vi "main.vi"() -> ()   [LabVIEW 2017]
uses:
  <vilib>/Platform/TimedLoop/XDataNode/wakeup.ctl
  <vilib>/Platform/TimedLoop/XDataNode/XDNodeRunTimeDep.lvlib
  <vilib>/Platform/TimedLoop/XDataNode/nitl_modes.ctl
  <vilib>/Platform/TimedLoop/XDataNode/timing_clust.ctl
  <vilib>/Platform/TimedLoop/XDataNode/XDataNode.xnode
  <vilib>/xnet/xnet.llb/XNET Frame Type CAN.ctl
  <vilib>/xnet/xnet.llb/XNET Frame CAN.ctl
  <vilib>/rvi/interface/nirviReadWriteControl/nirviReadWriteControl.xnode
  FPGA Bitfiles/FPGA.ctl
  FPGA Bitfiles/PVemulator_FPGATarget2_IpDFT-only-DC2x9_aEit3VyAdvg.lvbitx
  <vilib>/xnet/xnet.llb/XNET Write (Frame CAN).vi
  <vilib>/xnet/xnet.llb/XNET Read (Frame CAN).vi
  NiFpgaLv.dll
  <vilib>/Utility/error.llb/Error Cluster From Error Code.vi
  <vilib>/rvi/errors/niLvFpgaAdjustHostInterfaceError.vi
  General purpose/measurements.ctl
panel:
  out "Numeric":i32
  in  "Meas":T1
  out "V_PV1":dbl
  out "Ok to Close Contactor":bool
  out "CAN frame":T2 {"payload" format="%x"; "timestamp" format="%<%.7X\n%x>T"; "type" items=["CAN Data"=0, "CAN Remote"=1, "CAN Bus Error"=2, "CAN 2.0 Data"=8, "CAN FD Data"=16, "CAN FD+BRS Data"=24, "J1939 Data"=192, "Delay"=224, "Log Trigger"=225, "Start Trigger"=226]; "identifier" format="%x"}
  out "Vdc DCLink":dbl
  out "RPi Monitoring":bool
  out "Pconv":dbl
  out "Alarm list":string
  in  "Meas period [ms]":i64=10
  in  "newfile":bool
  in  "Log period [ms]":i64=1000
  out "Con_State":u8(ring) items=["Idle"=0, "Busy"=1, "Wait4srcON"=2, "Ready"=3, "Injecting"=6]
  in  "Emergency":bool
  in  "p_sp":dbl
  in  "Conv":T4
  in  "CAN [ms]":i64=1
  out "full":bool
  out "neg":bool
  out "precharge":bool
  out "CAN with Conv":bool
  out "Measurements":bool
  in  "Shutdwn":bool
  in  "Clear":bool
  in  "SEND sp":bool
  in  "Start":bool
  out "Error":u8(ring) items=["None", "Converter (water/temp/desat)", "Overvalue (hardware detected)", "Internal DC bus low", "Internal DC bus high", "External source DC low", "External source DC high", "Grid present (while VSC)", "Grid voltage out of range", "Grid frequency out of range", "No Grid (while CSC)", "Cannot clear (Manual clear needed)", "User Emergency", "Latch-up (Restart BBX)"]
  out "logging":bool
  in  "main stop":bool
  # "Resource agent: PV emulator x2 + Battery"
  # "PV Emulator for a DC grid"
  # "package identifiers:\n1xx PV emulator\n2xx PV emulator\n3xx PV emulator \n4xx battery\n\nx0x send from agent to resource\nx00 Power setpoints\nx01 Measurements\nx02 status\n          = [0; clear; 0; 0; 0; off; emergence; start]\n\n \n\nx1x send from resource to agent\nx10 Power measurements\nx11 Measurements\nx12 status\n          = [state; error; alarm; full; precharge; neg; 0; 0]"
  # "State:"
  # "DC +"
  # "DC -"
  # "CONVERTER CONTROL"
  # "PV"
  # "SETPOINTS"
  # "DC"
  # "DC"
  # "R"
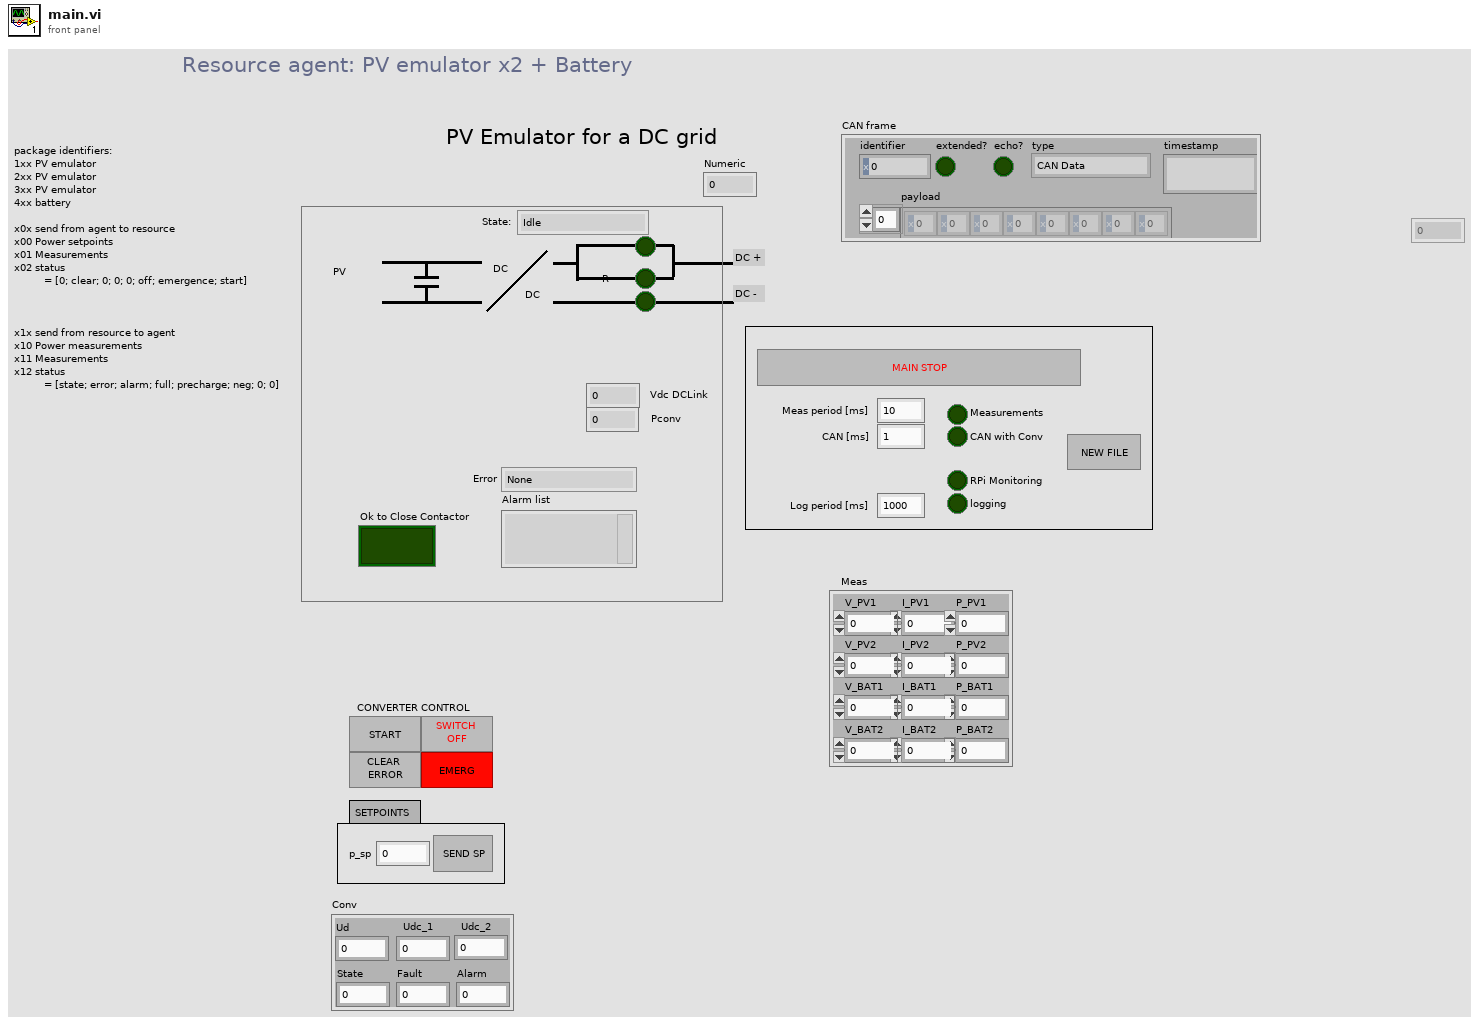
[diagram p1: front panel]
types:
  T1 = typedef "measurements.ctl" = cluster{"V_PV1":dbl, "I_PV1":dbl, "V_PV2":dbl, "I_PV2":dbl, "P_PV2":dbl, "V_BAT1":dbl, "I_BAT1":dbl, "P_BAT1":dbl, "V_BAT2":dbl, "I_BAT2":dbl, "P_BAT2":dbl, "P_PV1":dbl}
  T2 = typedef "XNET Frame CAN.ctl" = cluster{"timestamp":timestamp, "payload":u8[], "identifier":u32, "type":T3, "extended?":bool, "echo?":bool}
  T3 = typedef "XNET Frame Type CAN.ctl" = u8
  T4 = cluster{"Ud":dbl, "State":dbl, "Fault":dbl, "Alarm":dbl, "Udc_1":dbl, "Udc_2":dbl}
  T5 = typedef "FPGA.ctl" = refnum<k20>
  T6 = cluster{"Frame In":refnum<k21>, "Frame Out":refnum<k21>}
  T7 = typedef "XDNodeRunTimeDep.lvlib/timing_clust.ctl" = cluster{"Expected End [f-1]":u64, "Actual End [f-1]":u64, "Finished Late? [f-1]":bool, "Expected End [i-1]":u64, "Actual End [i-1]":u64, "Finished Late? [i-1]":bool, "Expected Start [i]":u64, "Actual Start [i]":u64, "Expected Start [f]":u64, "Actual Start [f]":u64, "Source Name":string, "Structure Name":string, "Period":i64, "Deadline":i64, "Offset":i64, "Start":i64, "Priority":i32, "Timeout":i32, "Mode":T8, "Wakeup Reason":T9, "Error":errorcluster, "Source Type":string, "Secondary Source Type":string, "Global End Time":u64, "Global Start Time":u64, "Frame Duration":u64, "Iteration Duration":u64, "Assigned CPU":i32, "I/O Scan Engine Mode":u32}
  T8 = typedef "XDNodeRunTimeDep.lvlib/nitl_modes.ctl" = enum32{"No Change", "Process missed periods, maintain original phase", "Discard missed periods, maintain original phase", "Process missed periods, ignore original phase", "Discard missed periods, ignore original phase"}
  T9 = typedef "XDNodeRunTimeDep.lvlib/wakeup.ctl" = enum32{"Normal", "Aborted", "Asynchronous wakeup", "Timing source error", "Timed loop error", "Timeout"}
  T10 = cluster{"V_PV1":dbl, "I_PV1":dbl, "V_PV2":dbl, "I_PV2":dbl, "P_PV2":dbl, "V_BAT1":dbl, "I_BAT1":dbl, "P_BAT1":dbl, "V_BAT2":dbl, "I_BAT2":dbl, "P_BAT2":dbl, "P_PV1":dbl}
  T11 = cluster{"date string":string, "time string":string, "V_PV1":dbl, "I_PV1":dbl, "P_PV1":dbl, "V_PV2":dbl, "I_PV2":dbl, "P_PV2":dbl, "V_BAT1":dbl, "I_BAT1":dbl, "P_BAT1":dbl, "V_BAT2":dbl, "I_BAT2":dbl, "P_BAT2":dbl}
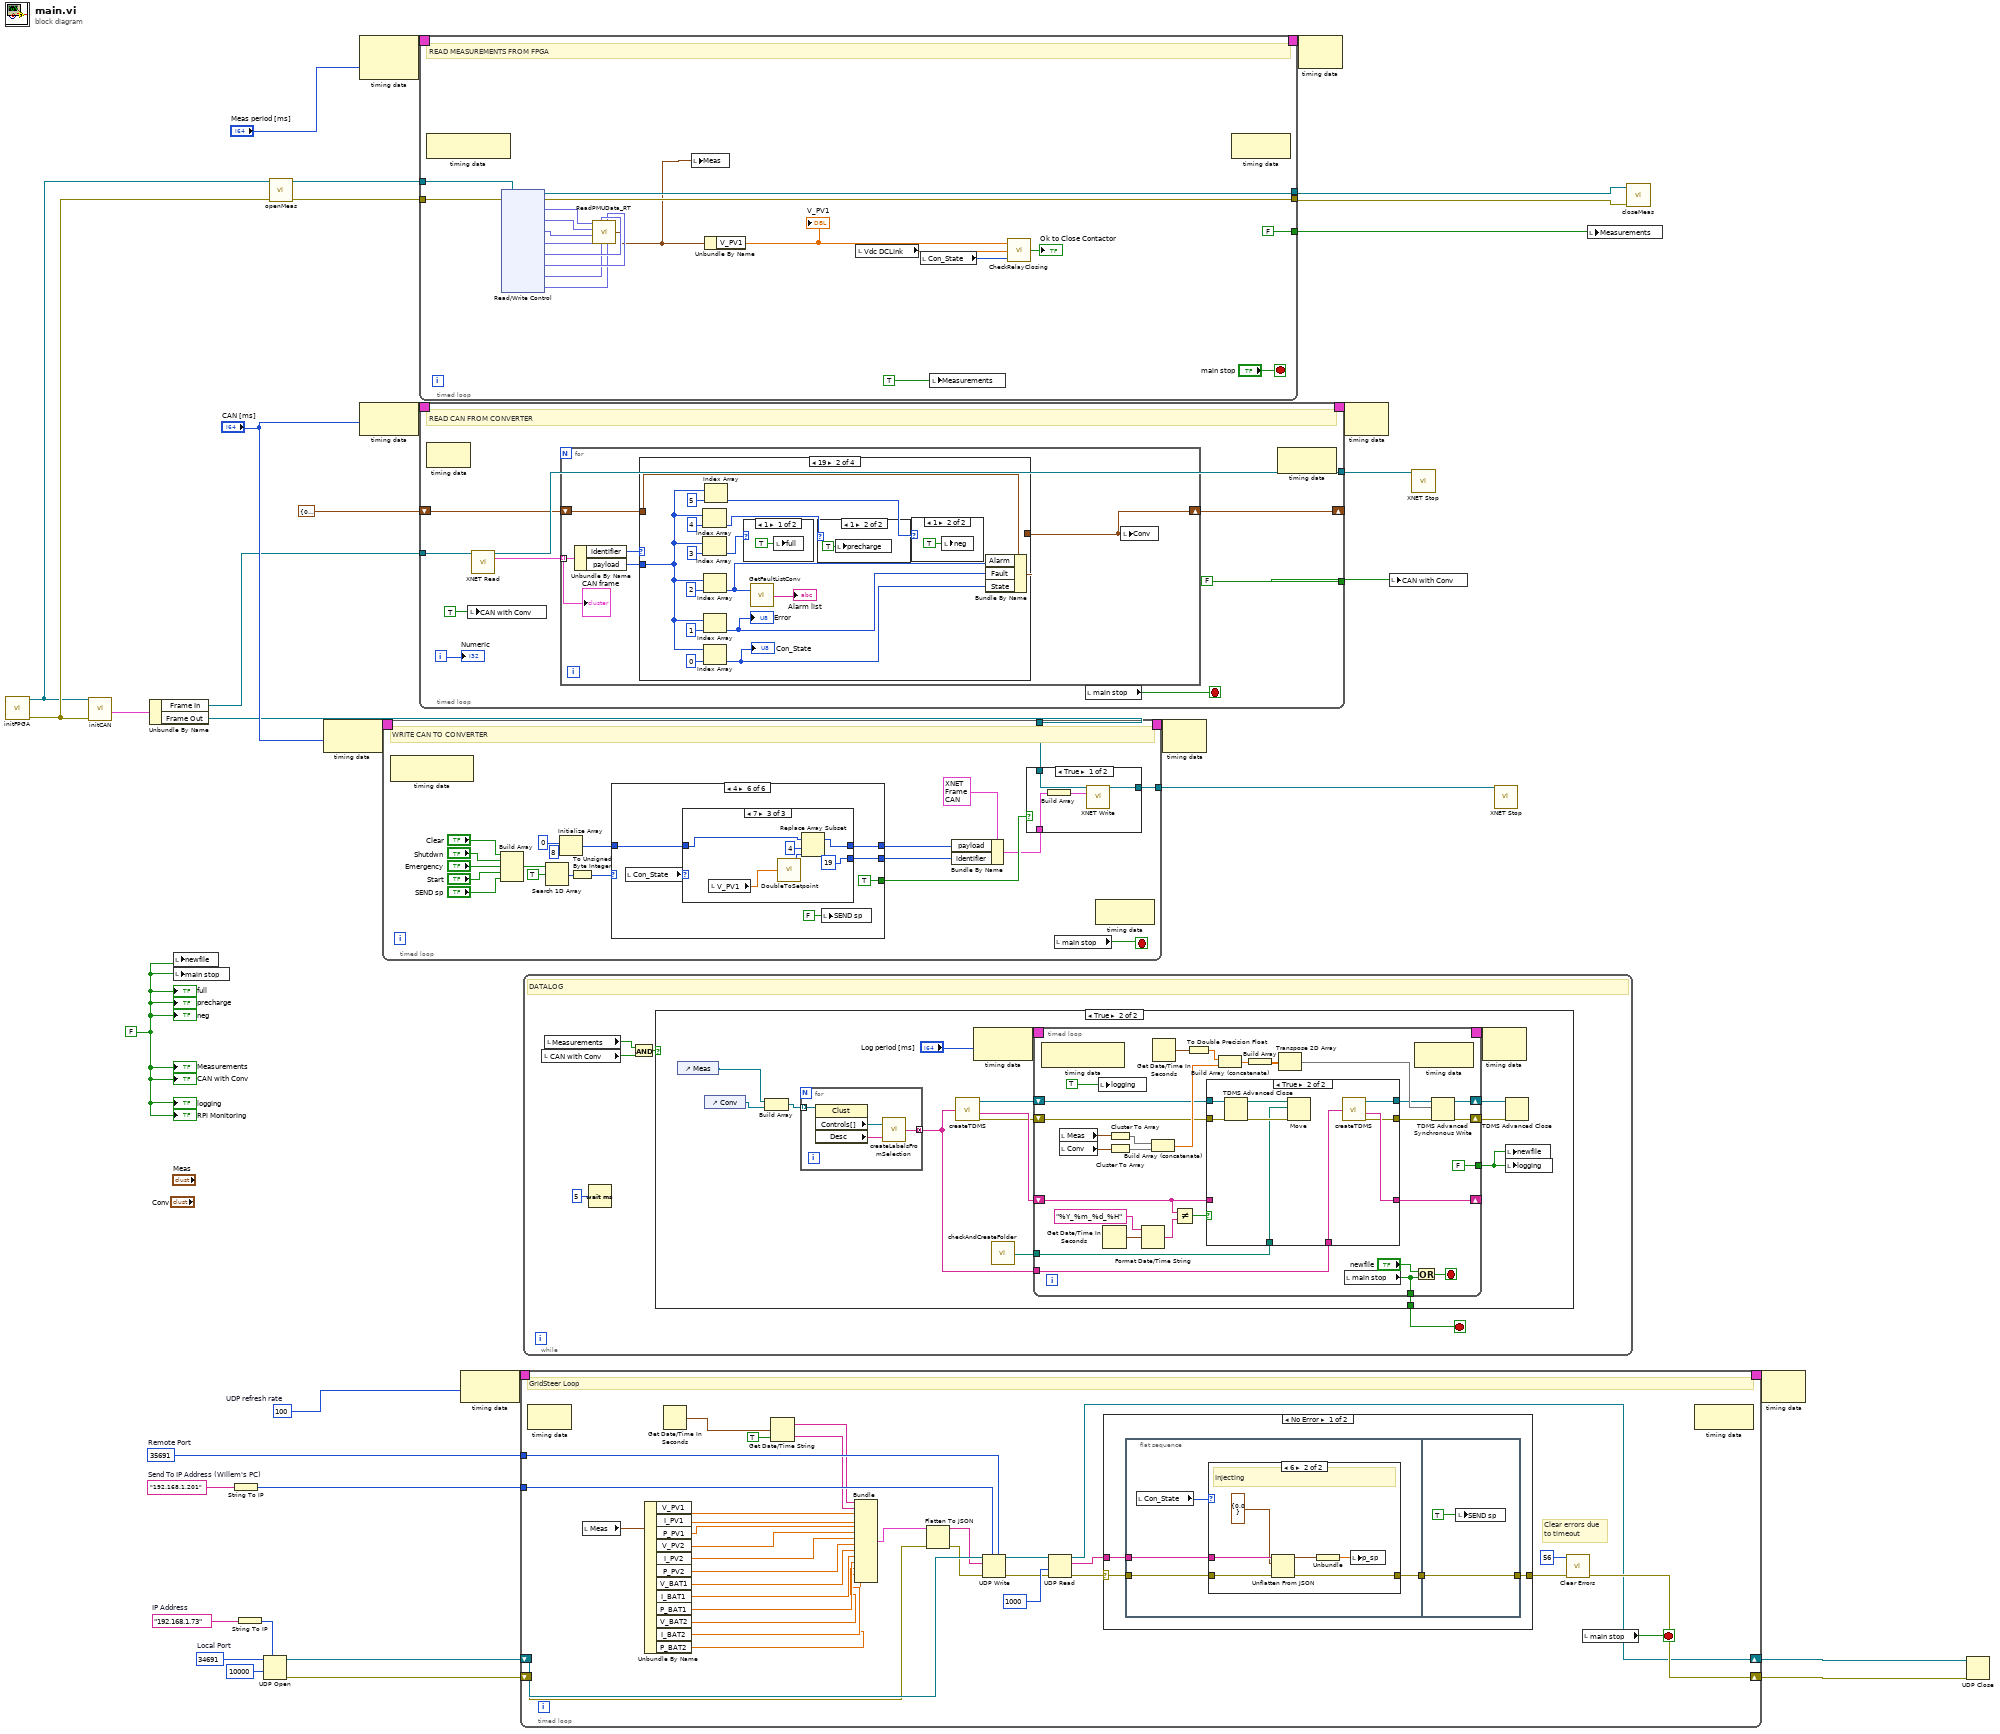
[diagram p0: block diagram]
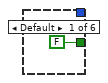
[diagram p7: hidden frame]
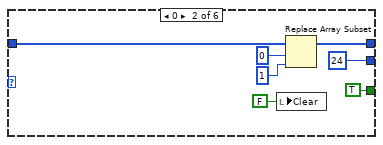
[diagram p8: hidden frame]
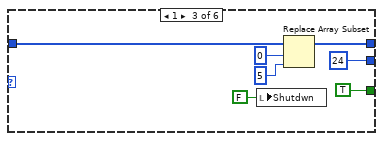
[diagram p9: hidden frame]
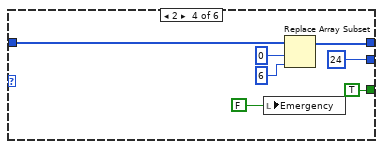
[diagram p10: hidden frame]
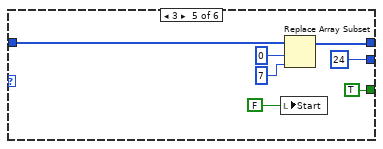
[diagram p11: hidden frame]
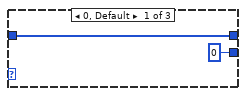
[diagram p12: hidden frame]
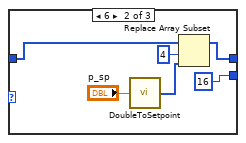
[diagram p13: hidden frame]
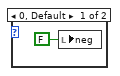
[diagram p15: hidden frame]
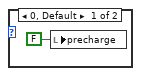
[diagram p16: hidden frame]
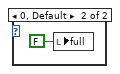
[diagram p17: hidden frame]
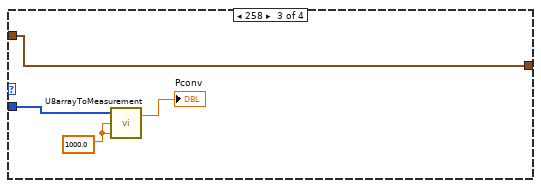
[diagram p18: hidden frame]
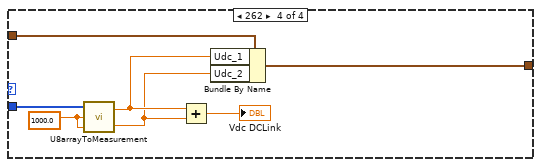
[diagram p19: hidden frame]
diagram:
  w5 = i64 100  # UDP refresh rate
  w10 = u16 34691  # Local Port
  w11 = "192.168.1.73"  # IP Address
  w1 = u16 35691  # Remote Port
  w9 = "192.168.1.201"  # Send To IP Address (Willem's PC)
  w17 = FALSE
  n1 = call "initFPGA.vi"() -> ("FPGA VI Reference Out"=w16:T5, "error out"=w18:errorcluster)  [unwired: 4 in]
  n2 = call "initCAN.vi"("error in"=w18, "FPGA VI (in)"=w16) -> ("CAN"=w31:T6)  [unwired: 3 in, 2 out]
  n3 = Unbundle By Name(w31) -> ("Frame In"=w21:refnum<k21>, "Frame Out"=w20:refnum<k21>)
  n4 = local write "newfile"(w17) -> ()
  n5 = local write "main stop"(w17) -> ()
  n6 = String To IP(1:w9) -> (0:w2:u32)
  n7 = String To IP(1:w11) -> (0:w12:u32)
  n8 = UDP Open(7:w12, 9:10000 ("timeout ms (25000)"), 11:w10) -> (port=w4:refnum<k16>, 0:w3:errorcluster)  [unwired: 2 in, 1 out]
  n9 = call "openMeas.vi"("error in"=w18, "FPGA VI (in)"=w16) -> ("error out"=w25:errorcluster, "FPGA VI (out)"=w26:T5)  [unwired: 7 in, 1 out]
  n10 = node-c288("CAN [ms]") -> (w33:T7)
  n11 = node-c288("Meas period [ms]") -> (w37:T7)  [unwired: 1 in]
  n12 = node-c288("CAN [ms]") -> (w35:T7)
  n13 = timed-loop {
    tunnel: w20 -> [w49]
    tunnel: [w48] -> w29
    timing: w33 -> [_]
    timing-out: [_] -> w32
    stop <- w47 stop-if-true
    # "WRITE CAN TO CONVERTER"
    n14 = node-c288() -> ()  [unwired: 1 in, 1 out]
    n15 = Build Array("Clear", "Shutdwn", "Emergency", "Start", "SEND sp") -> (w46:bool[])
    n16 = Search 1D Array(1D array=w46, element=TRUE) -> (index of element=w40:i32)  [unwired: 1 in]
    n17 = Initialize Array(u8 0, 8 ("dimension size")) -> (w55:u8[])
    n18 = To Unsigned Byte Integer(number=w40) -> (unsigned 8bit integer=w44:u8)
    n19 = case shown="4" w44 {
      tunnel: [_ w70 w77 w83 w90 w98] -> w54
      tunnel: [_ u32 24 ("identifier") u32 24 ("identifier") u32 24 ("identifier") u32 24 ("identifier") w95] -> w53
      tunnel: w55 -> [_ w68 w76 w84 w91 w93]
      tunnel: [FALSE TRUE TRUE TRUE TRUE TRUE] -> w51
      frame Default {
      }
      frame 0 {
        n20 = local write "Clear"(FALSE ("Clear")) -> ()
        n21 = Replace Array Subset(array=w68, new element=u8 1 ("new element/subarray"), index=0) -> (w70:u8[])
      }
      frame 1 {
        n22 = local write "Shutdwn"(FALSE ("Shutdwn")) -> ()
        n23 = Replace Array Subset(array=w76, new element=u8 5 ("new element/subarray"), index=0) -> (w77:u8[])
      }
      frame 2 {
        n24 = local write "Emergency"(FALSE ("Idc cmd")) -> ()
        n25 = Replace Array Subset(array=w84, new element=u8 6 ("new element/subarray"), index=0) -> (w83:u8[])
      }
      frame 3 {
        n26 = local write "Start"(FALSE ("Idc cmd")) -> ()
        n27 = Replace Array Subset(array=w91, new element=u8 7 ("new element/subarray"), index=0) -> (w90:u8[])
      }
      frame 4 {
        n28 = local read "Con_State"() -> (w94:u8)
        n29 = case shown="7" w94 {
          tunnel: [w100 w104 w110] -> w98
          tunnel: [u32 0 ("identifier") u32 16 ("identifier") u32 19 ("identifier")] -> w95
          tunnel: w93 -> [w100 w102 w107]
          frame 0, Default {
          }
          frame 6 {
            n30 = call "DoubleToSetpoint.vi"("Double"="p_sp") -> ("SP"=w103:u8[])
            n31 = Replace Array Subset(array=w102, new element=w103, index=4) -> (w104:u8[])
          }
          frame 7 {
            n32 = local read "V_PV1"() -> (w111:dbl)
            n33 = call "DoubleToSetpoint.vi"("Double"=w111) -> ("SP"=w109:u8[])
            n34 = Replace Array Subset(array=w107, new element=w109, index=4) -> (w110:u8[])
          }
        }
        n35 = local write "SEND sp"(FALSE ("SEND sp")) -> ()
      }
    }
    n36 = Bundle By Name(cluster=T2 {"timestamp"=timestamp(0 s since 1904-01-01), "payload"=[], "identifier"=0, "type"=0, "extended?"=FALSE, "echo?"=FALSE} ("CAN frame 3"), "payload"=w54, "identifier"=w53) -> (w50:T2)
    n37 = case shown="True" w51 {
      tunnel: w50 -> [w63 _]
      tunnel: w49 -> [w61 _]
      tunnel: [w60 _] -> w48
      frame True {
        n38 = Build Array(w63) -> (w62:T2[])
        n39 = call-poly <vilib>:"XNET Write.vi"("session in"=w61, "data"=w62) -> ("session out"=w60:refnum<k21>)  [unwired: 12 in, 1 out]
      }
      frame False {
      }
    }
    n40 = local read "main stop"() -> (w47:bool)
    n41 = node-c288() -> ()  [unwired: 1 in, 1 out]
  }
  n42 = timed-loop {
    timing: w37 -> [_]
    timing-out: [_] -> w36
    tunnel: w26 -> [w124]
    tunnel: [w125] -> w24
    tunnel: [w126] -> w23
    tunnel: [FALSE] -> w27
    tunnel: w25 -> [w123]
    stop <- "main stop" stop-if-true
    # "READ MEASUREMENTS FROM FPGA"
    n43 = node-c288() -> ()  [unwired: 1 in, 1 out]
    n44 = xnode "Read/Write Control"("FPGA VI Reference In"=w124, "error in"=w123) -> ("FPGA VI Reference Out"=w125:T5, "error out"=w126:errorcluster, "V_PV1"=w122:fxp<+,20,5>, "I_PV1"=w121:fxp<+,20,5>, "V_PV2"=w120:fxp<+/-,20,5>, "I_PV2"=w119:fxp<+/-,20,5>, "V_BAT1"=w118:fxp<+/-,20,5>, "I_BAT1"=w117:fxp<+,20,5>, "V_BAT2"=w116:fxp<+,20,5>, "I_BAT2"=w115:fxp<+/-,20,5>)
    n45 = call "ReadPMUData_RT.vi"("I_BAT2"=w115, "I_BAT1"=w117, "V_BAT2"=w116, "I_PV2"=w119, "V_PV2"=w120, "V_BAT1"=w118, "I_PV1"=w121, "V_PV1"=w122) -> ("measurements"=w113:T10)  [unwired: 2 in]
    n46 = local write "Meas"(w113) -> ()
    n47 = Unbundle By Name(w113) -> ("V_PV1"=w114:dbl)
    "V_PV1" <- w114
    n48 = local read "Vdc DCLink"() -> (w128:dbl)
    n49 = local read "Con_State"() -> (w127:u8)
    n50 = local write "Measurements"(TRUE) -> ()
    n51 = call "CheckRelayClosing.vi"("Converter State"=w127, "Vdc DC Link"=w128, "Vdc Battery"=w114) -> ("Ok to Close Contactor"=→"Ok to Close Contactor":bool)
    n52 = node-c288() -> ()  [unwired: 1 in, 1 out]
  }
  n53 = timed-loop {
    timing: w35 -> [_]
    timing-out: [_] -> w34
    tunnel: w21 -> [w135]
    tunnel: [w142] -> w30
    shift-right: [w137] -> _
    shift-left: T4 {"Ud"=0.0, "State"=0.0, "Fault"=0.0, "Alarm"=0.0, "Udc_1"=0.0, "Udc_2"=0.0} ("Conv") -> [w141]
    tunnel: [FALSE ("stop CAN")] -> w19
    i -> [w136]
    stop <- w140 stop-if-true
    # "READ CAN FROM CONVERTER"
    n54 = node-c288() -> ()  [unwired: 1 in, 1 out]
    n55 = local write "CAN with Conv"(TRUE) -> ()
    n56 = call-poly <vilib>:"XNET Read.vi"("session in"=w135) -> ("session out"=w142:refnum<k21>, "data"=w143:T2[])  [unwired: 11 in, 2 out]
    n57 = for {
      tunnel: w143 -> [w146] mode=indexing
      shift-right: [w144] -> w137
      shift-left: w141 -> [w145]
      n58 = Unbundle By Name(w146) -> ("identifier"=w148:u32, "payload"=w147:u8[])
      n59 = case shown="19" w148 {
        tunnel: w147 -> [_ w152 w175 w181]
        tunnel: w145 -> [w149 w162 w172 w179]
        tunnel: [w149 w161 w172 w180] -> w144
        frame 0, Default {
        }
        frame 25 {
          n60 = Index Array(array=w152, index=4) -> (element=w151:u8)
          n61 = Index Array(array=w152, index=3) -> (element=w156:u8)
          n62 = Index Array(array=w152, index=2) -> (element=w159:u8)
          n63 = Index Array(array=w152, index=1) -> (element=w160:u8)
          "Error" <- w160
          n64 = Index Array(array=w152, index=0) -> (element=w157:u8)
          "Con_State" <- w157
          n65 = Index Array(array=w152, index=5) -> (element=w150:u8)
          n66 = case shown="1" w156 {
            frame 1 {
              n67 = local write "full"(TRUE ("full")) -> ()
            }
            frame 0, Default {
              n68 = local write "full"(FALSE ("full")) -> ()
            }
          }
          n69 = call "GetFaultListConv.vi"("Fault message"=w159) -> ("Fault list"=→"Alarm list":string)  [unwired: 1 in]
          n70 = case shown="1" w151 {
            frame 0, Default {
              n71 = local write "precharge"(FALSE ("precharge")) -> ()
            }
            frame 1 {
              n72 = local write "precharge"(TRUE ("precharge")) -> ()
            }
          }
          n73 = case shown="1" w150 {
            frame 0, Default {
              n74 = local write "neg"(FALSE ("neg")) -> ()
            }
            frame 1 {
              n75 = local write "neg"(TRUE ("neg")) -> ()
            }
          }
          n76 = Bundle By Name(cluster=w162, "Alarm"=w159, "Fault"=w160, "State"=w157) -> (w161:T4)
        }
        frame 258 {
          w173 = 1000.0 ("factor 1")
          n77 = call "U8arrayToMeasurement.vi"("factor 2"=w173, "factor 1"=w173, "payload"=w175) -> ("Meas 1"=→"Pconv":dbl)  [unwired: 1 out]
        }
        frame 262 {
          w182 = 1000.0 ("factor 1")
          n78 = call "U8arrayToMeasurement.vi"("factor 2"=w182, "factor 1"=w182, "payload"=w181) -> ("Meas 2"=w177:dbl, "Meas 1"=w178:dbl)
          n79 = Add(x=w178, y=w177) -> (x+y=→"Vdc DCLink":dbl)
          n80 = Bundle By Name(cluster=w179, "Udc_1"=w178, "Udc_2"=w177) -> (w180:T4)
        }
      }
      n81 = local write "Conv"(w144) -> ()
      "CAN frame" <- w146
    }
    n82 = local read "main stop"() -> (w140:bool)
    n83 = node-c288() -> ()  [unwired: 1 in, 1 out]
    "Numeric" <- w136
  }
  n84 = node-c288(w5) -> (w14:T7)
  n85 = timed-loop {
    timing: w14 -> [_]
    timing-out: [_] -> w13
    shift-right: [w202] -> w8
    shift-left: w4 -> [w218]
    shift-right: [w208] -> w7
    shift-left: w3 -> [w215]
    tunnel: w2 -> [w212]
    tunnel: w1 -> [w211]
    stop <- w210 stop-if-true
    # "Clear errors due\nto timeout"
    # "GridSteer Loop"
    n86 = node-c288() -> ()  [unwired: 1 in, 1 out]
    n87 = local read "Meas"() -> (w196:T1)
    n88 = Unbundle By Name(w196) -> ("V_PV1"=w217:dbl, "I_PV1"=w216:dbl, "P_PV1"=w195:dbl, "V_PV2"=w194:dbl, "I_PV2"=w192:dbl, "P_PV2"=w191:dbl, "V_BAT1"=w190:dbl, "I_BAT1"=w189:dbl, "P_BAT1"=w188:dbl, "V_BAT2"=w187:dbl, "I_BAT2"=w186:dbl, "P_BAT2"=w185:dbl)
    n89 = Get Date/Time In Seconds() -> (seconds since 1Jan1904=w200:timestamp)
    n90 = Get Date/Time String(seconds (now)=w200, want seconds? (F)=TRUE) -> (date string=w199:string, time string=w198:string)  [unwired: 1 in]
    n91 = Bundle("date string"=w199, "time string"=w198, "V_PV1"=w217, "I_PV1"=w216, "P_PV1"=w195, "V_PV2"=w194, "I_PV2"=w192, "P_PV2"=w191, "V_BAT1"=w190, "I_BAT1"=w189, "P_BAT1"=w188, "V_BAT2"=w187, "I_BAT2"=w186, "P_BAT2"=w185) -> (w193:T11)  [unwired: 1 in]
    n92 = Flatten To JSON(anything=w193, error in (no error)=w215) -> (JSON string=w213:string, 11:w214:errorcluster)  [unwired: 1 in]
    n93 = UDP Write(address=w212, port or service name=w211, connection ID=w218, data in=w213, 8:w214) -> (error out=w204:errorcluster, 3:w203:refnum<k16>)  [unwired: 1 in]
    n94 = UDP Read(connection ID=w203, timeout ms (25000)=1000, 8:w204) -> (data out=w207:string, error out=w206:errorcluster, 3:w202:refnum<k16>)  [unwired: 1 in, 2 out]
    n95 = case shown="No Error" w206 {
      selector: w206 -> [w221 w236]
      tunnel: w207 -> [w222 _]
      tunnel: [w219 w236] -> w201
      frame No Error {
        n96 = flat-sequence {
          tunnel: w222 -> [w225]
          tunnel: w221 -> [w224]
          tunnel: [w223] -> w220
          tunnel: w220 -> [w235]
          tunnel: [w235] -> w219
          frame #0 {
            n97 = local read "Con_State"() -> (w226:u8)
            n98 = case shown="6" w226 {
              tunnel: w225 -> [_ w233]
              tunnel: w224 -> [w227 w232]
              tunnel: [w227 w231] -> w223
              frame Default {
              }
              frame 6 {
                # "Injecting"
                n99 = Unflatten From JSON(JSON string=w233, type and defaults=cluster{"P":dbl} {"P"=0.0} ("output cluster"), error in (no error)=w232) -> (value=w230:cluster{"P":dbl}, error out=w231:errorcluster)  [unwired: 4 in]
                n100 = Unbundle(w230) -> ("P"=w229:dbl)
                n101 = local write "p_sp"(w229) -> ()
              }
            }
          }
          frame #1 {
            n102 = local write "SEND sp"(TRUE ("SEND sp")) -> ()
          }
        }
      }
      frame Error {
      }
    }
    n103 = call <vilib>:"Clear Errors.vi"("error in (no error)"=w201, "specific error code to clear (0: all)"=56) -> ("error out"=w208:errorcluster)  [unwired: 4 in, 1 out]
    n104 = local read "main stop"() -> (w210:bool)
    n105 = node-c288() -> ()  [unwired: 1 in, 1 out]
  }
  n106 = while {
    stop <- w243 stop-if-true
    # "DATALOG"
    n107 = local read "CAN with Conv"() -> (w241:bool)
    n108 = local read "Measurements"() -> (w240:bool)
    n109 = Wait (ms)(milliseconds to wait=u32 5) -> ()  [unwired: 1 out]
    n110 = Compound Arithmetic op=AND(w240, w241) -> (w239:bool)
    n111 = case shown="True" w239 {
      selector: w239 -> [w244 _]
      tunnel: [w244 w257] -> w243
      frame False {
      }
      frame True {
        n112 = control-ref of="Meas"() -> (w245:refnum<vi>)
        n113 = control-ref of="Conv"() -> (w250:refnum<vi>)
        n114 = Build Array(w245, w250) -> (w249:refnum<vi>[])
        n115 = for {
          tunnel: [w261] -> w248 mode=concatenating
          tunnel: w249 -> [w260] mode=indexing
          n116 = property class="Clust"(reference=w260) -> ("Controls[]"=w263:refnum<vi>[], "Desc"=w262:string)  [unwired: 1 in, 2 out]
          n117 = call "createLabelsFromSelection.vi"("log_from"=w262, "Controls[]"=w263) -> ("labels_to_log"=w261:string[])
        }
        n118 = call "createTDMS.vi"("channel name(s)"=w248) -> ("Ref"=w246:refnum<k34>, "hour"=w252:string, "error out"=w247:errorcluster)  [unwired: 3 in]
        n119 = node-c288("Log period [ms]") -> (w259:T7)
        n120 = call "checkAndCreateFolder.vi"() -> ("dup path"=w251:path)  [unwired: 1 in]
        n121 = timed-loop {
          timing: w259 -> [_]
          timing-out: [_] -> w258
          tunnel: [w283] -> w257
          tunnel: [FALSE ("logging")] -> w253
          shift-right: [w274] -> _
          shift-left: w252 -> [w273]
          tunnel: w251 -> [w272]
          tunnel: w248 -> [w271]
          shift-right: [w284] -> w254
          shift-left: w247 -> [w265]
          shift-right: [w292] -> w255
          shift-left: w246 -> [w264]
          stop <- w286 stop-if-true
          n122 = node-c288() -> ()  [unwired: 1 in, 1 out]
          n123 = local read "Meas"() -> (w270:T1)
          n124 = local read "Conv"() -> (w269:T4)
          n125 = local write "logging"(TRUE ("logging")) -> ()
          n126 = Get Date/Time In Seconds() -> (seconds since 1Jan1904=w277:timestamp)
          n127 = Cluster To Array(cluster=w270) -> (array=w268:dbl[])
          n128 = Cluster To Array(cluster=w269) -> (array=w267:dbl[])
          n129 = Format Date/Time String(time format string (%c)="%Y_%m_%d_%H", seconds (now)=w277) -> (date/time string=w275:string)  [unwired: 1 in]
          n130 = Build Array (concatenate)(w268, w267) -> (w266:dbl[])
          n131 = Get Date/Time In Seconds() -> (seconds since 1Jan1904=w288:timestamp)
          n132 = Not Equal?(x=w273, y=w275) -> (x != y?=w276:bool)
          n133 = To Double Precision Float(number=w288) -> (double precision float=w287:dbl)
          n134 = case shown="True" w276 {
            tunnel: w264 -> [w295 w304]
            tunnel: [w295 w298] -> w280
            tunnel: w265 -> [w294 w303]
            tunnel: [w294 w296] -> w279
            tunnel: [w293 w297] -> w274
            tunnel: w273 -> [w293 _]
            tunnel: w272 -> [_ w300]
            tunnel: w271 -> [_ w299]
            frame False {
            }
            frame True {
              n135 = TDMS Advanced Close(8:w303, 11:w304) -> (0:w302:errorcluster, 3:w301:path)  [unwired: 2 in]
              n136 = Move(source path=w301, error in=w302, 10:w300) -> ()  [unwired: 2 in, 3 out]
              n137 = call "createTDMS.vi"("channel name(s)"=w299) -> ("Ref"=w298:refnum<k34>, "hour"=w297:string, "error out"=w296:errorcluster)  [unwired: 3 in]
            }
          }
          n138 = Build Array (concatenate)(w287, w266) -> (w291:dbl[])
          n139 = Build Array(w291) -> (w290:dbl[][])
          n140 = Transpose 2D Array(2D array=w290) -> (transposed array=w289:dbl[][])
          n141 = local read "main stop"() -> (w283:bool)
          n142 = node-c288() -> ()  [unwired: 1 in, 1 out]
          n143 = Or(x="newfile", y=w283) -> (x .or. y?=w286:bool)
          n144 = TDMS Advanced Synchronous Write(8:w279, 10:w289, 11:w280) -> (0:w284:errorcluster, 3:w292:refnum<k34>)
        }
        n145 = node-c288(w258) -> ()  [unwired: 1 out]
        n146 = TDMS Advanced Close(8:w254, 11:w255) -> ()  [unwired: 2 in, 2 out]
        n147 = local write "newfile"(w253) -> ()
        n148 = local write "logging"(w253) -> ()
      }
    }
  }
  n149 = node-c288(w32) -> ()  [unwired: 1 out]
  n150 = node-c288(w36) -> ()  [unwired: 1 out]
  n151 = node-c288(w34) -> ()  [unwired: 1 out]
  n152 = local write "CAN with Conv"(w19) -> ()
  n153 = call <vilib>:"XNET Stop.vi"("session in"=w30) -> ()  [unwired: 13 in, 2 out]
  n154 = call <vilib>:"XNET Stop.vi"("session in"=w29) -> ()  [unwired: 13 in, 2 out]
  n155 = local write "Measurements"(w27) -> ()
  n156 = call "closeMeas.vi"("error in (no error)"=w23, "FPGA VI (in) 2"=w24) -> ()  [unwired: 10 in]
  n157 = node-c288(w13) -> ()  [unwired: 1 out]
  n158 = UDP Close(connection ID=w8, 8:w7) -> ()  [unwired: 2 out]
  "full" <- w17
  "precharge" <- w17
  "Measurements" <- w17
  "CAN with Conv" <- w17
  "neg" <- w17
  "logging" <- w17
  "RPi Monitoring" <- w17
